vi "Tank Fills and Empties Automatically.vi"() -> ()   [LabVIEW 2016]
panel:
  out "Tank":dbl(slide) scale=0.0..100.0
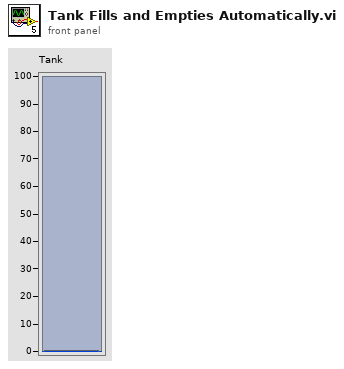
[diagram p1: front panel]
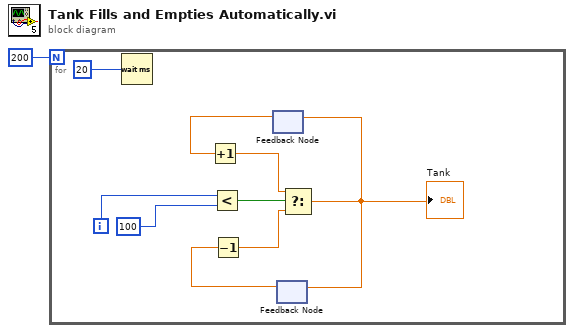
[diagram p0: block diagram]
diagram:
  n1 = for {
    N: 200 ("Numeric") -> [_]
    i -> [w5]
    n2 = Wait (ms)(milliseconds to wait=20) -> ()  [unwired: 1 out]
    n3 = Less?(x=w5, y=100) -> (x < y?=w8:bool)
    n4 = feedback #1() -> (w3:dbl)  [unwired: 1 in]
    n5 = Increment(x=w3) -> (x+1=w7:dbl)
    n6 = feedback #2() -> (w4:dbl)  [unwired: 1 in]
    n7 = Decrement(x=w4) -> (x-1=w6:dbl)
    n8 = Select(t=w7, s=w8, f=w6) -> (s? t:f=w2:dbl)
    "Tank" <- w2
    n9 = feedback-in #1(w2) -> ()
    n10 = feedback-in #2(w2) -> ()
  }
